vi "dategmt_timestamp.vi"(11 "String":string) -> (3 "time stamp":timestamp)   [LabVIEW 2011]
panel:
  out "trimmed string":string
  out "error out":errorcluster
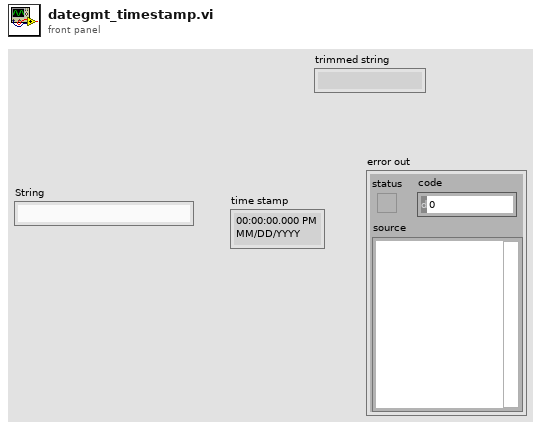
[diagram p1: front panel]
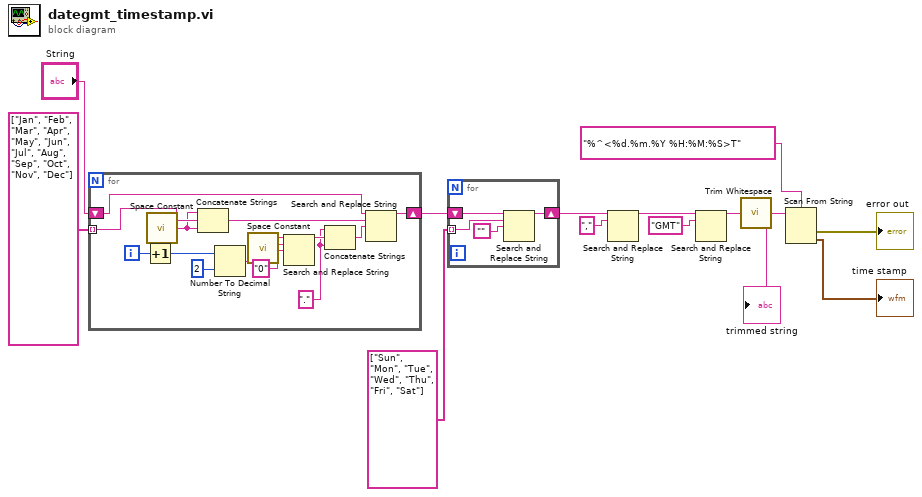
[diagram p0: block diagram]
diagram:
  n1 = for {
    tunnel: string[] ["Jan", "Feb", "Mar", "Apr", "May", "Jun", "Jul", "Aug", "Sep", "Oct", "Nov", "Dec"] -> [w19] mode=indexing
    shift-right: [w20] -> w7
    shift-left: "String" -> [w27]
    i -> [w26]
    w15 = "." ("string")
    n2 = Increment(x=w26) -> (x+1=w25:i32)
    n3 = call <vilib>:"Space Constant.vi"() -> ("String"=w18:string)
    n4 = Concatenate Strings(w18, w19, w18) -> (w17:string)
    n5 = Number To Decimal String(number=w25, width (-)=i16 2) -> (decimal integer string=w23:string)
    n6 = call <vilib>:"Space Constant.vi"() -> ("String"=w22:string)
    n7 = Search and Replace String(input string=w23, search string=w22, replace string="0" ("replace string (\"\")")) -> (result string=w16:string)  [unwired: 5 in, 3 out]
    n8 = Concatenate Strings(w15, w16, w15) -> (w14:string)
    n9 = Search and Replace String(input string=w27, search string=w17, replace string=w14) -> (result string=w20:string)  [unwired: 5 in, 3 out]
  }
  n10 = for {
    tunnel: string[] ["Sun", "Mon", "Tue", "Wed", "Thu", "Fri", "Sat"] -> [w30] mode=indexing
    shift-right: [w29] -> w6
    shift-left: w7 -> [w31]
    n11 = Search and Replace String(input string=w31, search string=w30, replace string="") -> (result string=w29:string)  [unwired: 5 in, 3 out]
  }
  n12 = Search and Replace String(input string=w6, search string=",") -> (result string=w4:string)  [unwired: 6 in, 3 out]
  n13 = Search and Replace String(input string=w4, search string="GMT") -> (result string=w2:string)  [unwired: 6 in, 3 out]
  n14 = call <vilib>:"Trim Whitespace.vi"("string"=w2) -> ("trimmed string"=w1:string)  [unwired: 1 in]
  "trimmed string" <- w1
  n15 = Scan From String(format string="%^<%d.%m.%Y %H:%M:%S>T" ("input string"), input string=w1) -> (error out=→"error out":errorcluster, output 1=→"time stamp":timestamp)  [unwired: 2 in, 3 out]
